vi "crio_FPGA_VCA_Sine_Sweep.vi"() -> ()   [LabVIEW 2019]
uses:
  <vilib>/rvi/Analysis/control/PID/Typedef/niFpgaPID_PIGains.ctl
  <vilib>/rvi/Analysis/control/PID/Typedef/niFpgaPID_ManualControl.ctl
  <vilib>/Platform/TimedLoop/XDataNode/timing_clust.ctl
  <vilib>/Platform/TimedLoop/XDataNode/nitl_modes.ctl
  <vilib>/Platform/TimedLoop/XDataNode/wakeup.ctl
  <vilib>/rvi/FXPMathLib/basic elements/FxpIntAccumulator/subVIs/nifxpmath_IntAccumulator_SimConfig.ctl
  <vilib>/rvi/FXPMathLib/FxpRectToPolar/subVIs/nifxpmath_RectToPolar_SimConfig.ctl
  <vilib>/rvi/Emulation/niFpgaSctlEmulationGetInTimedLoop.vi
  <vilib>/rvi/Emulation/niFpgaProcessEmulError.vi
  <vilib>/rvi/eio/common/nirviEmuTemplateMethod_errors.vi
  <vilib>/rvi/Emulation/niFpgaGetClockAttributes.vi
  <vilib>/rvi/Emulation/niFpgaEmulationReportErrorSimple.vi
  <vilib>/rvi/Emulation/niFpgaCriticalErrorInLSC.vi
  <vilib>/rvi/Analysis/common/codeGenErrors/XNode/niFpgaXNodeCodeGenErrorHandle.vi
  <vilib>/rvi/FXPMathLib/basic elements/FxpIntAccumulator/simVIs/DllFxpIntAccumulator_sub.vi
  <vilib>/rvi/FXPMathLib/FxpRectToPolar/simVIs/DllFxpRectToPolarTemp_sub.vi
  <vilib>/eio/EIOMethodNode/EIOMethodNode.xnode
  <vilib>/eio/EIONode/EIONode.xnode
  <vilib>/rvi/FXPMathLib/FxpInterpret/XNode/nifxpmath_Interpret.xnode
  <vilib>/rvi/FXPMathLib/FxpMul/XNode/nifxpmath_Multiplier.xnode
  <vilib>/rvi/FXPMathLib/FxpAdd/XNode/nifxpmath_Add.xnode
  <vilib>/rvi/Analysis/measure/mean-var-std/XNode/niFpgaMean-Var-Std.xnode
  <vilib>/platform/TimedLoop/XDataNode/XDataNode.xnode
  <vilib>/rvi/FXPMathLib/basic elements/FxpIntAccumulator/XNode/nifxpmath_IntAccumulator.xnode
  <vilib>/rvi/FXPMathLib/FxpRectToPolar/XNode/nifxpmath_RectToPolar.xnode
  <vilib>/rvi/FXPMathLib/sim/FxpSim.dll
  <vilib>/Platform/TimedLoop/XDataNode/XDNodeRunTimeDep.lvlib
  <vilib>/rvi/Analysis/control/PID/Typedef/niFpgaPID_OutputRange.ctl
  <vilib>/rvi/Analysis/control/PID/SubVIs/niFpgaPID_PIWrapper.vi
panel:
  in  "sweep frequency (periods/tick)":fxp<+,32,0>=1.25030055642128e-06
  out "sine out":i16
  out "sin_fxp":fxp<+/-,16,1>
  out "cos_fxp":fxp<+/-,16,1>
  out "cosine out":i16
  in  "Lock_loop_rate":u32 caption="Count(uSec)"
  in  "Lock_debug":bool
  out "magnitude":fxp<+,32,6>
  out "phase (pi)":fxp<+/-,16,2>
  out "output valid":bool
  out "sin*input":fxp<+/-,32,6>
  out "cos*input":fxp<+/-,32,6>
  out "lock_input":fxp<+/-,16,5>
  in  "sin_gain":fxp<+,32,1>=0.5
  in  "sin_offset":fxp<+/-,16,3>=0.5
  out "ControllerPWM Output":sgl
  in  "manual control":T1 {"manual input (0)" scale=-1.0..1.0}
  in  "setpoint":i32
  in  "gains":T2 {"proportional gain" step=0.125}
  in  "Debug: ConnectorA/DIO15":bool
  in  "Debug: ConnectorA/DIO14":bool
  in  "Encoder Debug":bool
  in  "Loop Timer DAQ":u32=1 caption="Loop Time(uSec)"
  in  "Position Reset":bool
  out "Position (Counts)":i32
  out "B":bool
  out "A":bool
  out "B'":bool
  out "A'":bool
  in  "Velocity Interval (uSec)":u32=1000
  out "Acceleration (Counts/Interval)":i32
  out "Velocity (Counts/Interval)":i32
  in  "stop":bool
  in  "DC PWM Period (microsec)":i16=50
  # "1Hz -> sweep frequency: 2.5e-8\n5H -> 1.25e-7"
  # "DRV8256 Specs:\n\n0 0: Brake Low\n1 1: Brake High\nPWM 0\n0 PWM"
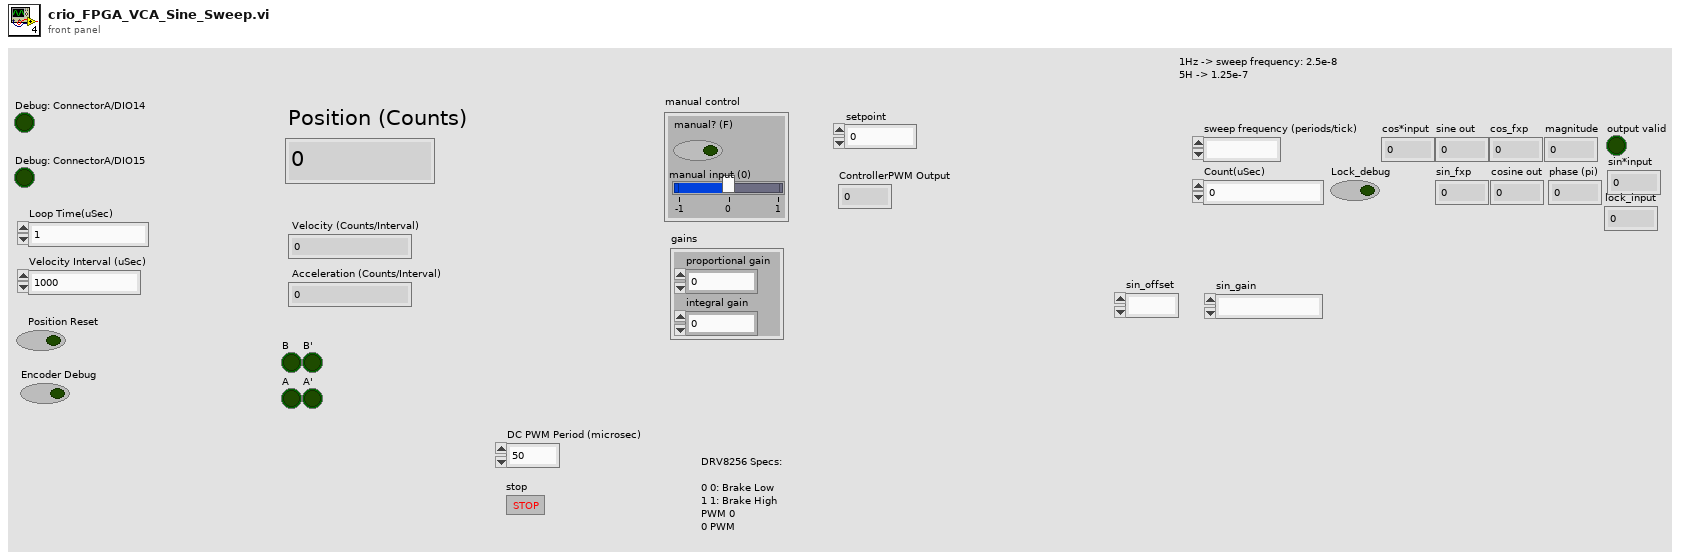
[diagram p1: front panel]
types:
  T1 = typedef "niFpgaPID_ManualControl.ctl" = cluster{"manual? (F)":bool, "manual input (0)":sgl}
  T2 = typedef "niFpgaPID_PIGains.ctl" = cluster{"proportional gain":sgl, "integral gain":sgl}
  T3 = typedef "niFpgaPID_OutputRange.ctl" = cluster{"output high (Inf)":sgl, "output low (-Inf)":sgl}
  T4 = typedef "XDNodeRunTimeDep.lvlib/timing_clust.ctl" = cluster{"Expected End [f-1]":u64, "Actual End [f-1]":u64, "Finished Late? [f-1]":bool, "Expected End [i-1]":u64, "Actual End [i-1]":u64, "Finished Late? [i-1]":bool, "Expected Start [i]":u64, "Actual Start [i]":u64, "Expected Start [f]":u64, "Actual Start [f]":u64, "Source Name":string, "Structure Name":string, "Period":i64, "Deadline":i64, "Offset":i64, "Start":i64, "Priority":i32, "Timeout":i32, "Mode":T5, "Wakeup Reason":T6, "Error":errorcluster, "Source Type":string, "Secondary Source Type":string, "Global End Time":u64, "Global Start Time":u64, "Frame Duration":u64, "Iteration Duration":u64, "Assigned CPU":i32, "I/O Scan Engine Mode":u32}
  T5 = typedef "XDNodeRunTimeDep.lvlib/nitl_modes.ctl" = enum32{"No Change", "Process missed periods, maintain original phase", "Discard missed periods, maintain original phase", "Process missed periods, ignore original phase", "Discard missed periods, ignore original phase"}
  T6 = typedef "XDNodeRunTimeDep.lvlib/wakeup.ctl" = enum32{"Normal", "Aborted", "Asynchronous wakeup", "Timing source error", "Timed loop error", "Timeout"}
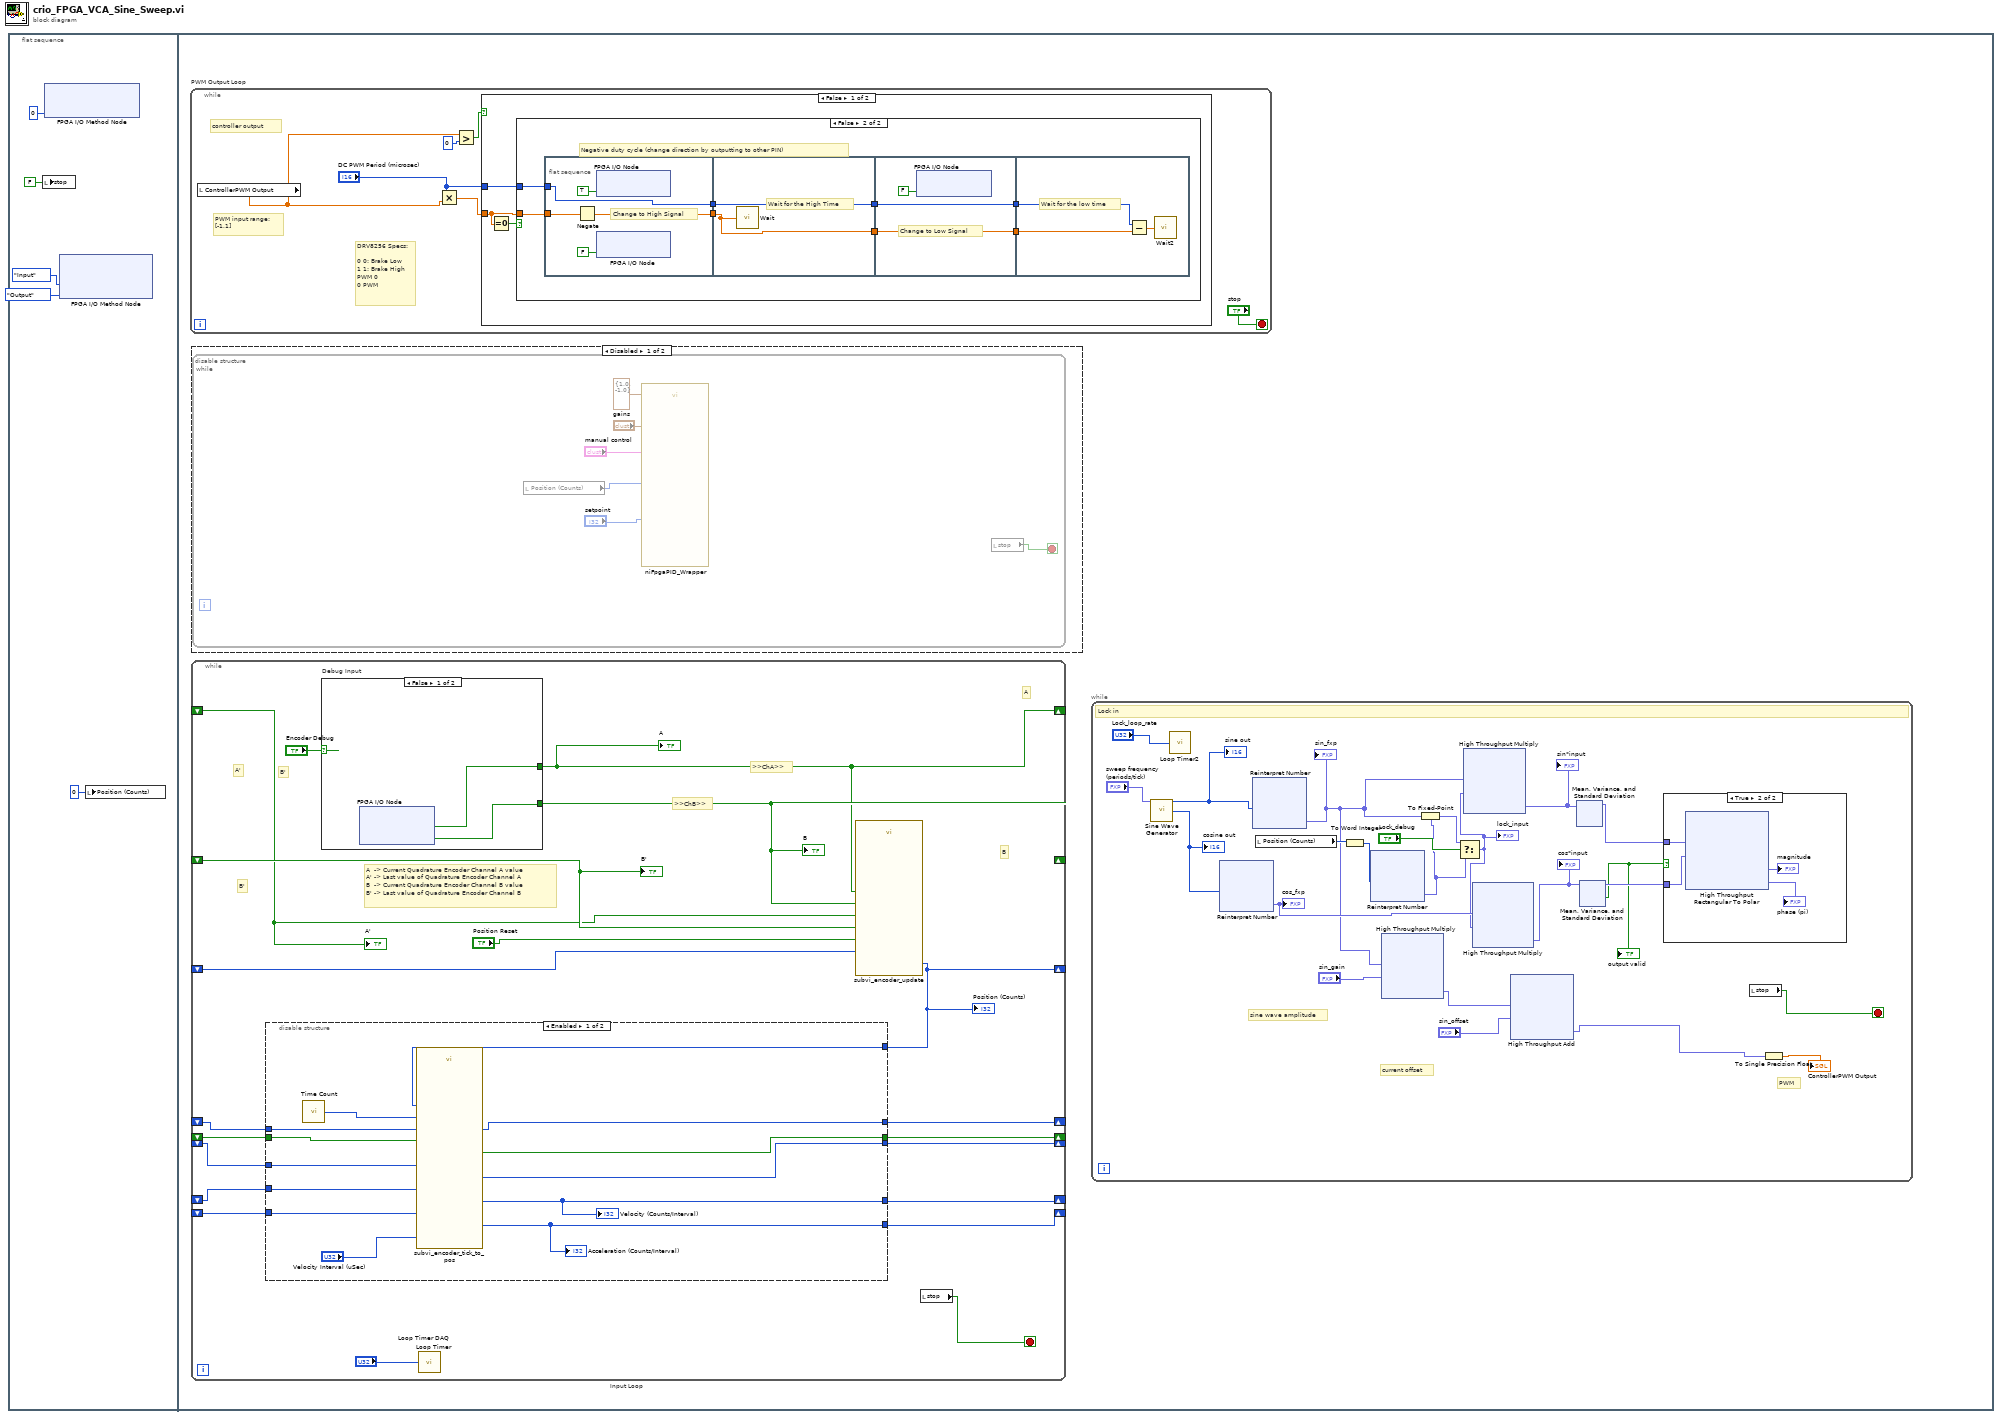
[diagram p0: block diagram]
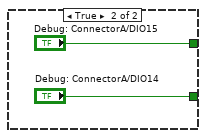
[diagram p5: hidden frame]
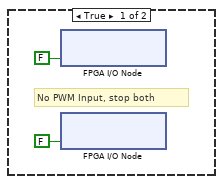
[diagram p6: hidden frame]
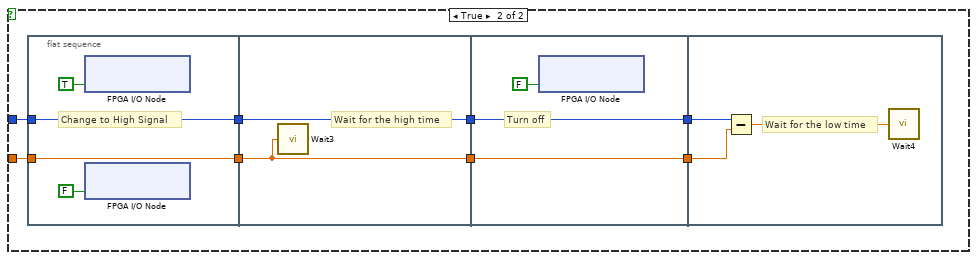
[diagram p7: hidden frame]
diagram:
  n1 = flat-sequence {
    frame #0 {
      n2 = local write "stop"(FALSE ("stop")) -> ()
      n3 = xnode "FPGA I/O Method Node"("Enable"=u8 0) -> ()  [unwired: 1 in, 1 out]
      n4 = xnode "FPGA I/O Method Node"("DIO 7:4"=enum8{"No Change", "Input", "Output"}."Input", "DIO 3:0"=enum8{"No Change", "Input", "Output"}."Output") -> ()  [unwired: 1 in, 1 out]
      n5 = local write "Position (Counts)"(0 ("Position (Counts)")) -> ()
    }
    frame #1 {
      n6 = while "PWM Output Loop" {
        stop <- "stop" stop-if-true
        # "PWM input range:\n[-1,1]"
        # "DRV8256 Specs:\n\n0 0: Brake Low\n1 1: Brake High\nPWM 0\n0 PWM"
        # "controller output"
        n7 = local read "ControllerPWM Output"() -> (w265:sgl)
        n8 = Multiply(x="DC PWM Period (microsec)", y=w265) -> (x*y=w267:sgl)
        n9 = Greater?(x=w265, y=i16 0) -> (0:w268:bool)
        n10 = case shown="False" w268 {
          tunnel: w267 -> [w273 w304]
          tunnel: "DC PWM Period (microsec)" -> [w271 w303]
          frame False {
            n11 = Equal To 0?(x=w273) -> (x = 0?=w272:bool)
            n12 = case shown="False" w272 {
              tunnel: w273 -> [_ w283]
              tunnel: w271 -> [_ w276]
              frame True {
                # "No PWM Input, stop both"
                n13 = xnode "FPGA I/O Node"("Mod1/DIO1"=FALSE) -> ()  [unwired: 1 in, 1 out]
                n14 = xnode "FPGA I/O Node"("Mod1/DIO0"=FALSE) -> ()  [unwired: 1 in, 1 out]
              }
              frame False {
                # "Negative duty cycle (change direction by outputting to other PIN)"
                n15 = flat-sequence {
                  tunnel: w283 -> [w286]
                  tunnel: [w285] -> w282
                  tunnel: [w284] -> w277
                  tunnel: w276 -> [w284]
                  tunnel: w282 -> [w290]
                  tunnel: [w290] -> w281
                  tunnel: [w289] -> w278
                  tunnel: w277 -> [w289]
                  tunnel: w281 -> [w292]
                  tunnel: [w292] -> w280
                  tunnel: [w291] -> w279
                  tunnel: w278 -> [w291]
                  tunnel: w280 -> [w296]
                  tunnel: w279 -> [w295]
                  frame #0 {
                    # "Change to High Signal"
                    n16 = Negate(x=w286) -> (-x=w285:sgl)
                    n17 = xnode "FPGA I/O Node"("Mod1/DIO1"=TRUE) -> ()  [unwired: 1 in, 1 out]
                    n18 = xnode "FPGA I/O Node"("Mod1/DIO0"=FALSE) -> ()  [unwired: 1 in, 1 out]
                  }
                  frame #1 {
                    # "Wait for the High Time"
                    n19 = call "Wait"("Count(uSec)"=w290) -> ()  [unwired: 1 out]
                  }
                  frame #2 {
                    # "Change to Low Signal"
                    n20 = xnode "FPGA I/O Node"("Mod1/DIO1"=FALSE) -> ()  [unwired: 1 in, 1 out]
                  }
                  frame #3 {
                    # "Wait for the low time"
                    n21 = Subtract(x=w295, y=w296) -> (x-y=w294:sgl)
                    n22 = call "Wait2"("Count(uSec)"=w294) -> ()  [unwired: 1 out]
                  }
                }
              }
            }
          }
          frame True {
            n23 = flat-sequence {
              tunnel: w304 -> [w305]
              tunnel: w303 -> [w306]
              tunnel: [w306] -> w300
              tunnel: [w305] -> w299
              tunnel: [w310] -> w301
              tunnel: w300 -> [w310]
              tunnel: w299 -> [w309]
              tunnel: [w309] -> w298
              tunnel: [w312] -> w302
              tunnel: w301 -> [w312]
              tunnel: w298 -> [w311]
              tunnel: [w311] -> w297
              tunnel: w302 -> [w316]
              tunnel: w297 -> [w314]
              frame #0 {
                # "Change to High Signal"
                n24 = xnode "FPGA I/O Node"("Mod1/DIO0"=TRUE) -> ()  [unwired: 1 in, 1 out]
                n25 = xnode "FPGA I/O Node"("Mod1/DIO1"=FALSE ("ConnectorB/DIO9")) -> ()  [unwired: 1 in, 1 out]
              }
              frame #1 {
                # "Wait for the high time"
                n26 = call "Wait3"("Count(uSec)"=w309) -> ()  [unwired: 1 out]
              }
              frame #2 {
                # "Turn off"
                n27 = xnode "FPGA I/O Node"("Mod1/DIO0"=FALSE) -> ()  [unwired: 1 in, 1 out]
              }
              frame #3 {
                # "Wait for the low time"
                n28 = Subtract(x=w316, y=w314) -> (x-y=w315:sgl)
                n29 = call "Wait4"("Count(uSec)"=w315) -> ()  [unwired: 1 out]
              }
            }
          }
        }
      }
      n30 = disable-structure shown="Disabled" {
        frame Disabled {
          n31 = while {
            stop <- w11 stop-if-true
            n32 = local read "Position (Counts)"() -> (w10:i32)
            n33 = call-poly <vilib>:"niFpgaPID_Wrapper.vi"("setpoint"="setpoint", "process variable"=w10, "manual control"="manual control", "gains"="gains", "output range"=T3 {"output high (Inf)"=1.0, "output low (-Inf)"=-1.0}) -> ()  [unwired: 8 in, 3 out]
            n34 = local read "stop"() -> (w11:bool)
          }
        }
        frame Enabled {
        }
      }
      n35 = while "Input Loop" {
        shift-right: [w241] -> _
        shift-left: _ -> [w244]
        shift-right: [w240] -> _
        shift-left: _ -> [w243]
        shift-right: [w236] -> _
        shift-left: _ -> [w242]
        shift-right: [w229] -> _
        shift-left: _ -> [w239]
        shift-right: [w230] -> _
        shift-left: _ -> [w238]
        shift-right: [w237] -> _
        shift-left: _ -> [w235]
        shift-right: [w234] -> _
        shift-left: _ -> [w233]
        shift-right: [w232] -> _
        shift-left: _ -> [w231]
        stop <- w228 stop-if-true
        # "B'"
        # ">>ChB>>"
        # ">>ChA>>"
        # "A'"
        # "A  -> Current Quadrature Encoder Channel A value\nA' -> Last value of Quadrature Encoder Channel A\nB  -> Current Quadrature Encoder Channel B value\nB' -> Last value of Quadrature Encoder Channel B"
        # "B'"
        # "B"
        # "A"
        n36 = case "Debug Input" shown="False" "Encoder Debug" {
          tunnel: [w262 "Debug: ConnectorA/DIO15"] -> w240
          tunnel: [w261 "Debug: ConnectorA/DIO14"] -> w241
          frame False {
            n37 = xnode "FPGA I/O Node"() -> ("Mod2/DIO0"=w262:bool, "Mod2/DIO1"=w261:bool)  [unwired: 2 in, 2 out]
          }
          frame True {
          }
        }
        "B" <- w241
        "A" <- w240
        n38 = call "Loop Timer"("Count(uSec)"="Loop Timer DAQ") -> ()  [unwired: 1 out]
        n39 = call "subvi_encoder_update.vi"("Position Reset"="Position Reset", "Tick'"=w242, "A"=w240, "B'"=w244, "A'"=w243, "B"=w241) -> ("Tick"=w236:i32)  [unwired: 5 in]
        "Position (Counts)" <- w236
        n40 = disable-structure shown="Enabled" {
          disable-tunnel: w239 -> [w259 _]
          disable-tunnel: w238 -> [w258 _]
          disable-tunnel: [w257 _] -> w237
          disable-tunnel: w236 -> [w256 _]
          disable-tunnel: w235 -> [w255 _]
          disable-tunnel: [w254 _] -> w234
          disable-tunnel: w233 -> [w253 _]
          disable-tunnel: [w252 _] -> w232
          disable-tunnel: w231 -> [w251 _]
          disable-tunnel: [w249 _] -> w230
          disable-tunnel: [w248 _] -> w229
          frame Enabled {
            n41 = call "Time Count"() -> ("Tick Count(uSec)"=w250:u32)
            n42 = call "subvi_encoder_tick_to_pos.vi"("Velocity Interval (uSec)"="Velocity Interval (uSec)", "Raw Tick"=w256, "Waited?'"=w253, "Tick Count(uSec)'"=w251, "p'"=w255, "Time Count"=w250, "a'"=w258, "v'"=w259) -> ("Waited?"=w254:bool, "Tick Count(uSec)"=w252:u32, "p"=w257:i32, "a"=w249:i32, "v"=w248:i32)  [unwired: 3 in]
            "Acceleration (Counts/Interval)" <- w249
            "Velocity (Counts/Interval)" <- w248
          }
          frame Disabled {
          }
        }
        n43 = local read "stop"() -> (w228:bool)
        "B'" <- w244
        "A'" <- w243
      }
      n44 = while {
        stop <- w12 stop-if-true
        # "PWM"
        # "current offset"
        # "sine wave amplitude"
        # "Lock in"
        n45 = call "Sine Wave Generator"("frequency (periods/tick)"="sweep frequency (periods/tick)") -> ("sine out"=w33:i16, "cosine out"=w32:i16)  [unwired: 13 in]
        "sine out" <- w33
        "cosine out" <- w32
        n46 = call "Loop Timer2"("Count(uSec)"="Lock_loop_rate") -> ()  [unwired: 1 out]
        n47 = xnode "Reinterpret Number"("x"=w32) -> ("y"=w29:fxp<+/-,16,1>)
        "cos_fxp" <- w29
        n48 = xnode "Reinterpret Number"("x"=w33) -> ("y"=w18:fxp<+/-,16,1>)
        "sin_fxp" <- w18
        n49 = local read "Position (Counts)"() -> (w31:i32)
        n50 = To Word Integer(number=w31) -> (16bit integer=w30:i16)
        n51 = xnode "Reinterpret Number"("x"=w30) -> ("y"=w25:fxp<+/-,16,5>)
        n52 = xnode ("High Throughput Multiply")("x"=w18, "y"="sin_gain") -> ("x*y"=w16:fxp<+/-,48,2>)
        n53 = To Fixed-Point(fixed-point type=w25, number=w18) -> (fixed-point=w26:fxp<+/-,16,5>)
        n54 = Select(t=w26, s="Lock_debug", f=w25) -> (s? t:f=w19:fxp<+/-,16,5>)
        "lock_input" <- w19
        n55 = xnode ("High Throughput Multiply")("x"=w18, "y"=w19) -> ("x*y"=w23:fxp<+/-,32,6>)
        "sin*input" <- w23
        n56 = xnode ("High Throughput Multiply")("x"=w29, "y"=w19) -> ("x*y"=w24:fxp<+/-,32,6>)
        "cos*input" <- w24
        n57 = xnode ("High Throughput Add")("x"=w16, "y"="sin_offset") -> ("x+y"=w14:fxp<+/-,50,4>)
        n58 = xnode "Mean, Variance, and Standard Deviation"("input data"=w23) -> ("mean"=w22:fxp<+/-,32,6>)  [unwired: 1 in, 1 out]
        n59 = xnode "Mean, Variance, and Standard Deviation"("input data"=w24) -> ("mean"=w21:fxp<+/-,32,6>, "output valid"=w20:bool)  [unwired: 1 in]
        "output valid" <- w20
        n60 = case shown="True" w20 {
          tunnel: w22 -> [_ w36]
          tunnel: w21 -> [_ w35]
          frame False {
          }
          frame True {
            n61 = xnode "High Throughput Rectangular To Polar"("x"=w36, "y"=w35) -> ("magnitude"=→"magnitude":fxp<+,32,6>, "phase (pi)"=→"phase (pi)":fxp<+/-,16,2>)
          }
        }
        n62 = local read "stop"() -> (w12:bool)
        n63 = To Single Precision Float(number=w14) -> (single precision float=→"ControllerPWM Output":sgl)
      }
    }
  }
